vi "setValue.vi"(8 "error in (no error)":errorcluster, 10 "value":variant, 11 "type in":refnum<class "type.lvclass">) -> (0 "error out":errorcluster, 3 "type out":refnum<class "type.lvclass">)   [LabVIEW 2015, in "type.lvclass"]
uses:
  type.lvclass
  type.lvclass/type.ctl
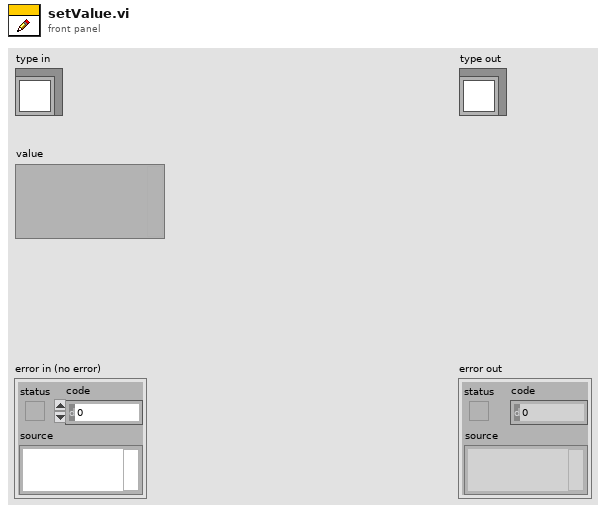
[diagram p1: front panel]
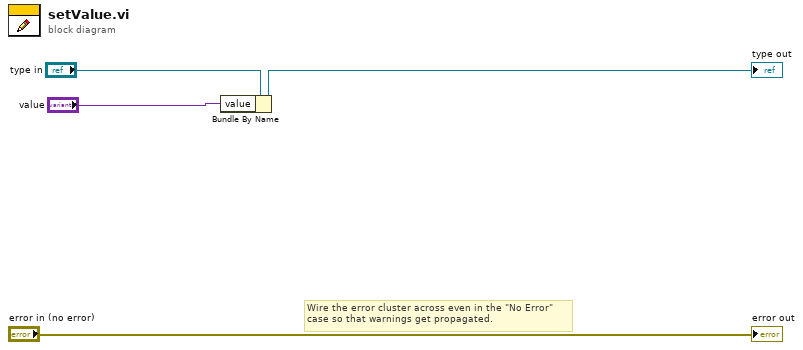
[diagram p0: block diagram]
diagram:
  # "Wire the error cluster across even in the \"No Error\"\ncase so that warnings get propagated."
  n1 = Bundle By Name(cluster="type in", "value"="value") -> (→"type out":refnum<class "type.lvclass">)
  "error out" <- "error in (no error)"
